vi "CONVERT ITEM DESCRIPTION DATA.vi"(11 "ITEM DESCRIPTION DATA IN":T2) -> (3 "ITEM DATA OUT":T1)   [LabVIEW 2019]
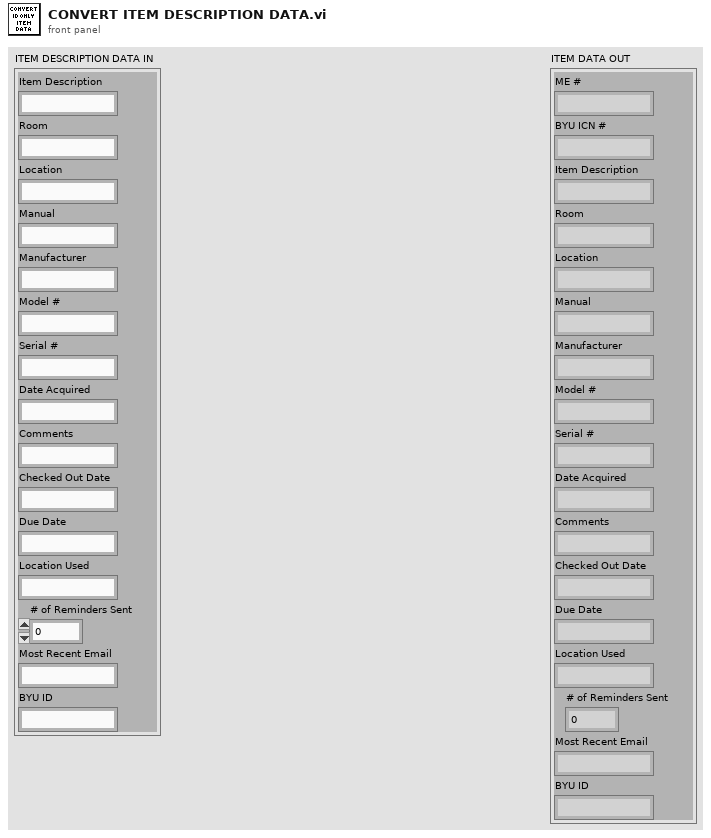
[diagram p1: front panel]
types:
  T1 = cluster{"ME #":string, "BYU ICN #":string, "Item Description":string, "Room":string, "Location":string, "Manual":string, "Manufacturer":string, "Model #":string, "Serial #":string, "Date Acquired":string, "Comments":string, "Checked Out Date":string, "Due Date":string, "Location Used":string, "# of Reminders Sent":i32, "Most Recent Email":string, "BYU ID":string}
  T2 = cluster{"Item Description":string, "Room":string, "Location":string, "Manual":string, "Manufacturer":string, "Model #":string, "Serial #":string, "Date Acquired":string, "Comments":string, "Checked Out Date":string, "Due Date":string, "Location Used":string, "# of Reminders Sent":i32, "Most Recent Email":string, "BYU ID":string}
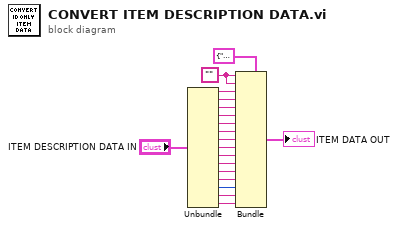
[diagram p0: block diagram]
diagram:
  w2 = ""
  n1 = Unbundle("ITEM DESCRIPTION DATA IN") -> ("Item Description"=w17:string, "Room"=w16:string, "Location"=w15:string, "Manual"=w14:string, "Manufacturer"=w13:string, "Model #"=w12:string, "Serial #"=w11:string, "Date Acquired"=w10:string, "Comments"=w9:string, "Checked Out Date"=w8:string, "Due Date"=w7:string, "Location Used"=w6:string, "# of Reminders Sent"=w3:i32, "Most Recent Email"=w5:string, "BYU ID"=w4:string)
  n2 = Bundle(cluster=T1 {"ME #"="", "BYU ICN #"="", "Item Description"="", "Room"="", "Location"="", "Manual"="", "Manufacturer"="", "Model #"="", "Serial #"="", "Date Acquired"="", "Comments"="", "Checked Out Date"="", "Due Date"="", "Location Used"="", "# of Reminders Sent"=0, "Most Recent Email"="", "BYU ID"=""} ("ITEM DATA"), "ME #"=w2, "BYU ICN #"=w2, "Item Description"=w17, "Room"=w16, "Location"=w15, "Manual"=w14, "Manufacturer"=w13, "Model #"=w12, "Serial #"=w11, "Date Acquired"=w10, "Comments"=w9, "Checked Out Date"=w8, "Due Date"=w7, "Location Used"=w6, "# of Reminders Sent"=w3, "Most Recent Email"=w5, "BYU ID"=w4) -> (→"ITEM DATA OUT":T1)
